vi "terminal point.vi"(2 "peaks/valleys":enum32{"Peaks", "Valleys"}(ring)=enum."Valleys", 3 "threshold":dbl caption="阈值" format="%0.2f", 4 "PD width":i32=3 caption="PD宽度" min=3, 5 "TDD filePath":path caption="TDD file Path") -> (0 "time low":dbl, 1 "time low index":dbl)   [LabVIEW 2011]
uses:
  <vilib>/Utility/file.llb/Read From Spreadsheet File (DBL).vi
  <vilib>/Analysis/NI_AAL_SigProc.lvlib
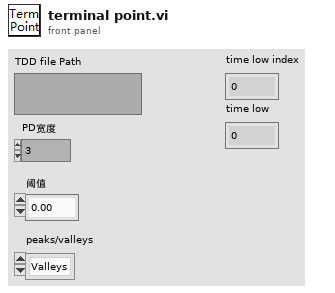
[diagram p1: front panel]
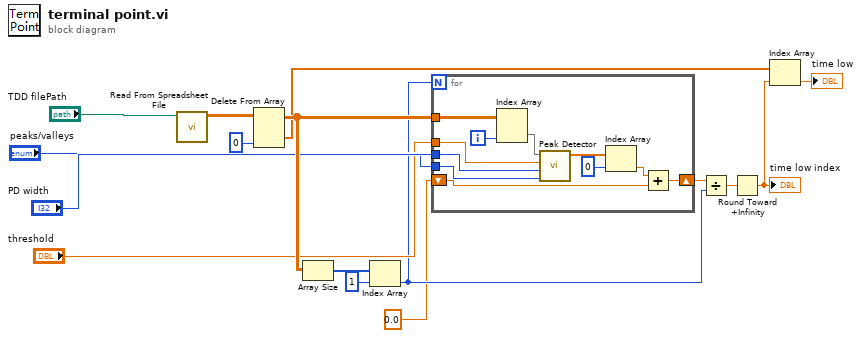
[diagram p0: block diagram]
diagram:
  n1 = call-poly <vilib>:"Read From Spreadsheet File.vi"("file path (dialog if empty)"="TDD filePath") -> ("all rows"=w14:dbl[][])  [unwired: 6 in, 4 out]
  n2 = Delete From Array(array=w14, index (col)=0 ("禁用的索引 (列)")) -> (deleted portion=w4:dbl[], array with subset deleted=w11:dbl[][])  [unwired: 2 in]
  n3 = Array Size(array=w11) -> (size(s)=w13:i32[])
  n4 = Index Array(array=w13, index=1 ("索引")) -> (element=w6:i32)
  n5 = for {
    N: w6 -> [_]
    tunnel: w11 -> [w27]
    tunnel: "PD width" -> [w24]
    tunnel: "peaks/valleys" -> [w23]
    tunnel: "threshold" -> [w22]
    shift-right: [w19] -> w7
    shift-left: 0.0 -> [w20]
    i -> [w26]
    n6 = Index Array(array=w27, index (col)=w26) -> (element=w25:dbl[])  [unwired: 1 in]
    n7 = call <vilib>:"Peak Detector.vi"("peaks/valleys"=w23, "width"=w24, "threshold"=w22, "X"=w25) -> ("Locations"=w21:dbl[])  [unwired: 3 in, 4 out]
    n8 = Index Array(array=w21, index=0 ("索引")) -> (element=w18:dbl)
    n9 = Add(x=w18, y=w20) -> (x+y=w19:dbl)
  }
  n10 = Divide(x=w7, y=w6) -> (x/y=w5:dbl)
  n11 = Round Toward +Infinity(x=w5) -> (ceil(x): smallest int >= x=w3:dbl)
  "time low index" <- w3
  n12 = Index Array(array=w4, index=w3) -> (element=→"time low":dbl)
